vi "Read Caller Enqueuer.vi"(11 "Actor":refnum<class "Actor.lvclass">) -> (2 "Caller Enqueuer":refnum<class "Message Enqueuer.lvclass">)   [LabVIEW 2013, in "Actor Framework.lvlib" / "Actor.lvclass"]
doc: "(<B>Filename</B>: Actor Framework.lvlib:Actor.lvclass:Read Caller Enqueuer.vi)\n\nReturns the reference the actor needs to send messages to its caller."
uses:
  <vilib>/ActorFramework/Actor/Actor.lvclass
  <vilib>/ActorFramework/Message Enqueuer/Message Enqueuer.lvclass
  <vilib>/ActorFramework/Actor/Actor.lvclass/Actor.ctl
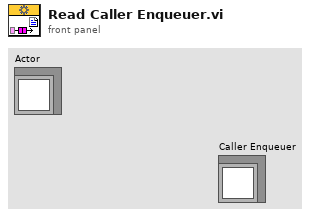
[diagram p1: front panel]
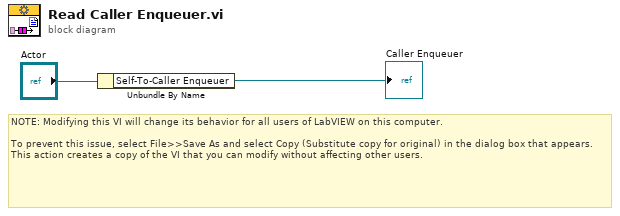
[diagram p0: block diagram]
diagram:
  # "NOTE: Modifying this VI will change its behavior for all users of LabVIEW on this computer.\n\nTo prevent this issue, select File>>Save As and select Copy (Substitute copy for original) in the dialog box that appears. This action creates a copy of the VI that you can modify without affecting other users."
  n1 = Unbundle By Name("Actor") -> ("Self-To-Caller Enqueuer"=→"Caller Enqueuer":refnum<class "Message Enqueuer.lvclass">)
